vi "Read_RobotLiftCommand.vi"(8 "error in (no error)":errorcluster, 11 "RobotLiftData in":refnum<class "RobotLiftData.lvclass">) -> (0 "error out":errorcluster, 2 "Robot Lift Command":T1, 3 "RobotLiftData out":refnum<class "RobotLiftData.lvclass">)   [LabVIEW 2017, in "RobotLiftData.lvclass"]
uses:
  RobotLiftData.lvclass
  Team-code/RobotLiftCommand.ctl
  Team-code/RunMode.ctl
  RobotLiftData.lvclass/RobotLiftData.ctl
  Team-code/RobotSubsystem.lvclass
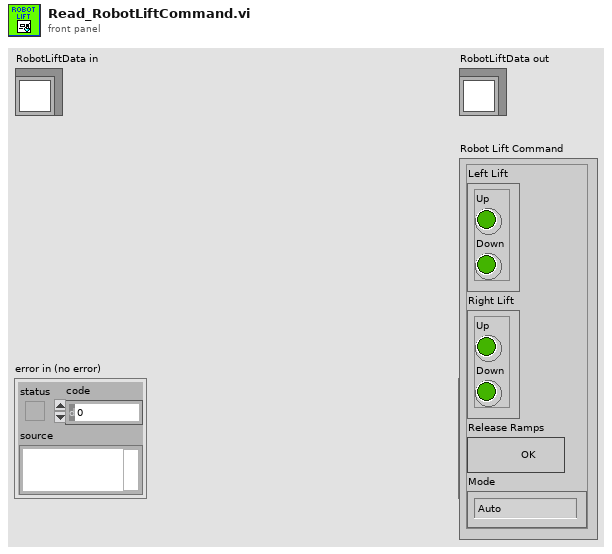
[diagram p1: front panel]
types:
  T1 = typedef "RobotLiftData.lvclass/RobotLiftCommand.ctl" = cluster{"Left Lift":cluster{"Up":bool, "Down":bool}, "Right Lift":cluster{"Up":bool, "Down":bool}, "Release Ramps":bool, "Mode":T2}
  T2 = typedef "RobotSubsystem.lvclass/RunMode.ctl" = enum16{"Auto", "Teleop", "Disabled"}
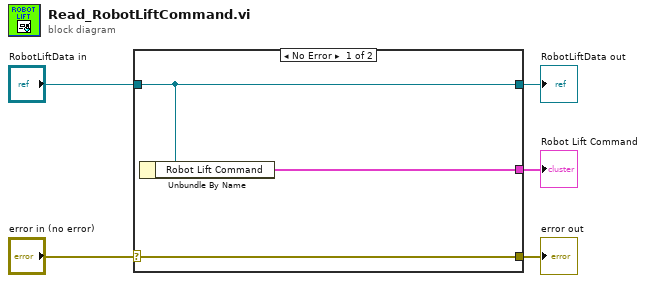
[diagram p0: block diagram]
diagram:
  n1 = case shown="No Error" "error in (no error)" {
    selector: "error in (no error)" -> [w8 w9]
    tunnel: [w8 w9] -> w4
    tunnel: [w7 w10] -> w2
    tunnel: "RobotLiftData in" -> [w7 w10]
    tunnel: [w6 _] -> w1
    frame No Error {
      n2 = Unbundle By Name(w7) -> ("Robot Lift Command"=w6:T1)
    }
    frame Error {
    }
  }
  "error out" <- w4
  "RobotLiftData out" <- w2
  "Robot Lift Command" <- w1
